vi "back-turn(SubVI).vi"(9 "Select Encoder":string, 10 "Select Channel":string, 11 "Motor Encoder Target":i32) -> ()   [LabVIEW 2016]
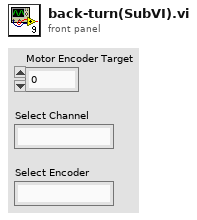
[diagram p1: front panel]
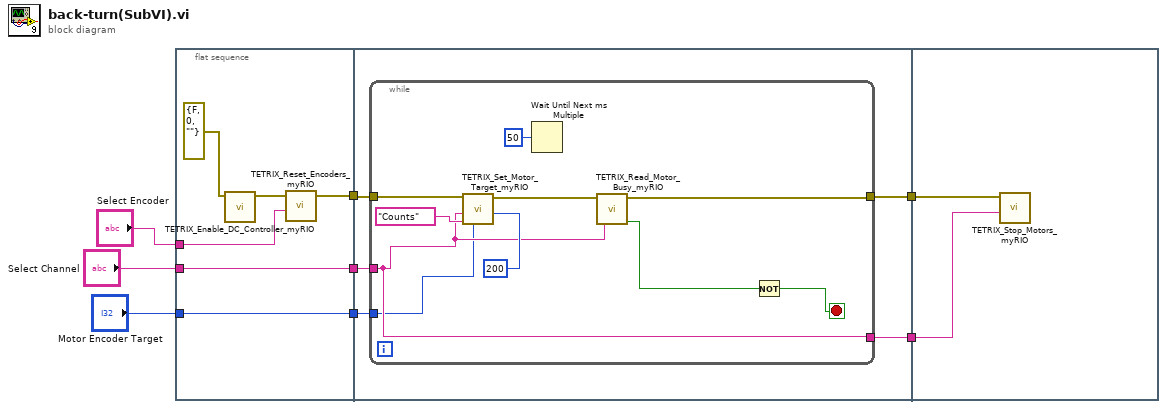
[diagram p0: block diagram]
diagram:
  n1 = flat-sequence {
    tunnel: [w13] -> w8
    tunnel: [w11] -> w7
    tunnel: "Select Channel" -> [w11]
    tunnel: "Select Encoder" -> [w10]
    tunnel: [w9] -> w6
    tunnel: "Motor Encoder Target" -> [w9]
    tunnel: w8 -> [w19]
    tunnel: [w18] -> w5
    tunnel: w7 -> [w17]
    tunnel: [w16] -> w4
    tunnel: w6 -> [w15]
    tunnel: w5 -> [w31]
    tunnel: w4 -> [w30]
    frame #0 {
      n2 = call <vilib>:"TETRIX_Enable_DC_Controller_myRIO.vi"("Error/Flow In"=errorcluster {"status"=FALSE, "code"=0, "source"=""}) -> ("Error/Flow Out"=w14:errorcluster)  [unwired: 6 in]
      n3 = call <vilib>:"TETRIX_Reset_Encoders_myRIO.vi"("Select Encoder"=w10, "Error/Flow In"=w14) -> ("Error/Flow Out"=w13:errorcluster)  [unwired: 5 in]
    }
    frame #1 {
      n4 = while {
        tunnel: w19 -> [w25]
        tunnel: [w26] -> w18
        tunnel: w17 -> [w22]
        tunnel: [w22] -> w16
        tunnel: w15 -> [w21]
        stop <- w20 stop-if-true
        n5 = call <vilib>:"TETRIX_Set_Motor_Target_myRIO.vi"("Motor Encoder Target"=w21, "Constant Speed (Degrees per Second)"=i16 200, "Encoder Units"="Counts", "Select Channel"=w22, "Error/Flow In"=w25) -> ("Error/Flow Out"=w27:errorcluster)  [unwired: 2 in]
        n6 = Wait Until Next ms Multiple(millisecond multiple=u32 50) -> ()  [unwired: 1 out]
        n7 = call <vilib>:"TETRIX_Read_Motor_Busy_myRIO.vi"("Select Channel"=w22, "Error/Flow In"=w27) -> ("Error/Flow Out"=w26:errorcluster, "Motor Busy?"=w24:bool)  [unwired: 4 in]
        n8 = Not(x=w24) -> (.not. x?=w20:bool)
      }
    }
    frame #2 {
      n9 = call <vilib>:"TETRIX_Stop_Motors_myRIO.vi"("Select Channel"=w30, "Error/Flow In"=w31) -> ()  [unwired: 5 in, 1 out]
    }
  }
